vi "Aquire Image.vi"(8 "error in (no error)":errorcluster, 10 "Stop":bool, 11 "Edmund Optics in":refnum<class "Edmund Optics.lvclass">) -> (0 "error out":errorcluster, 2 "Image Out":T1(plugin-control), 3 "Edmund Optics out":refnum<class "Edmund Optics.lvclass">)   [LabVIEW 2019, in "Edmund Optics.lvclass"]
uses:
  Edmund Optics.lvclass
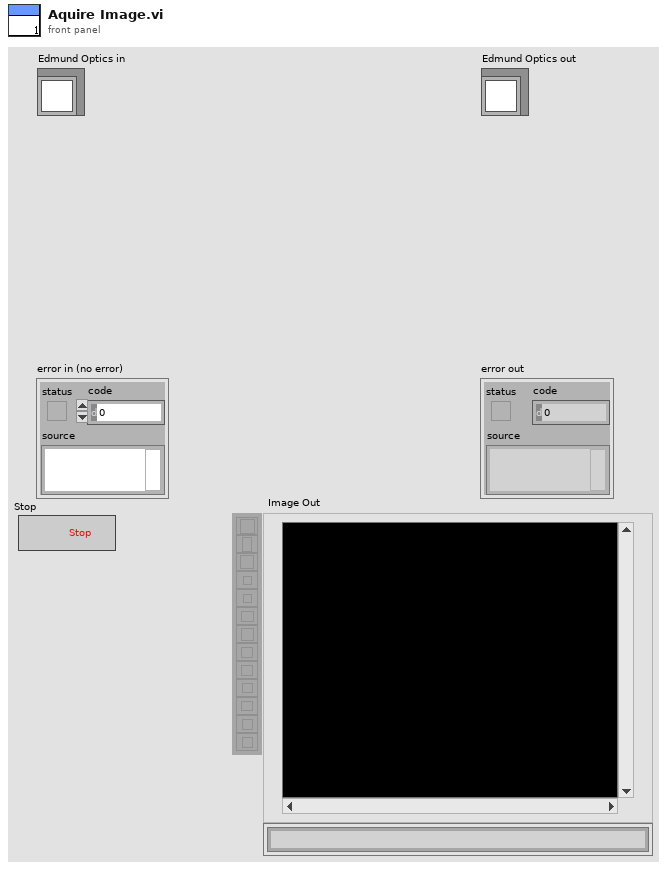
[diagram p1: front panel]
types:
  T1 = typedef "IMAQ Image.ctl" = refnum<image>
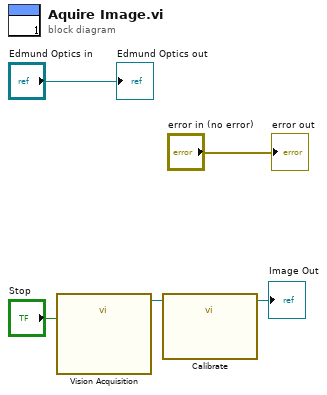
[diagram p0: block diagram]
diagram:
  n1 = call "Vision Acquisition"("Stop (F)"="Stop") -> ("Image Out"=w2:T1)  [unwired: 24 in, 2 out]
  n2 = call "Calibrate"("Image In"=w2) -> ("Image Out"=→"Image Out":T1)  [unwired: 25 in, 1 out]
  "error out" <- "error in (no error)"
  "Edmund Optics out" <- "Edmund Optics in"
